vi "LabVIEW Final Project read.vi"() -> ()   [LabVIEW 2022 SP3]
uses:
  <vilib>/sound2/lvsound2.llb/Sampling Mode.ctl
  <vilib>/Analysis/2dsp.llb/Real FFT.vi
  <vilib>/Analysis/baseanly.llb/Mean (DBL).vi
  <vilib>/sound2/lvsound2.llb/Sound Input Read (DBL).vi
  <vilib>/measure/matone.llb/Extract Multiple Tone Information 1 Chan.vi
  <vilib>/Utility/file.llb/Read Delimited Spreadsheet (DBL).vi
  <vilib>/Analysis/NI_AALPro.lvlib
  <vilib>/measure/NI_MAPro.lvlib
  <vilib>/Analysis/NI_AALBase.lvlib
panel:
  in  "stop":bool
  out "Average Percent Difference from Phase":dbl
  out "Average Percent Difference from Frequency":dbl
  out "Average Percent Difference from Amplitude":dbl format="%#_10g"
  out "On if same voice, Off if different":bool
  out "multiple tone information":T1(array[cluster]) {"detected phase (deg)" format="%_6g"; "detected amplitude" format="%_6p"; "detected frequency" format="%_6p"}
  out "Spectrum":dbl[](graph)
  out "Original":dbl[](graph)
  in  "Press to take input":bool
  # "Now I need to change Sensitivity Values"
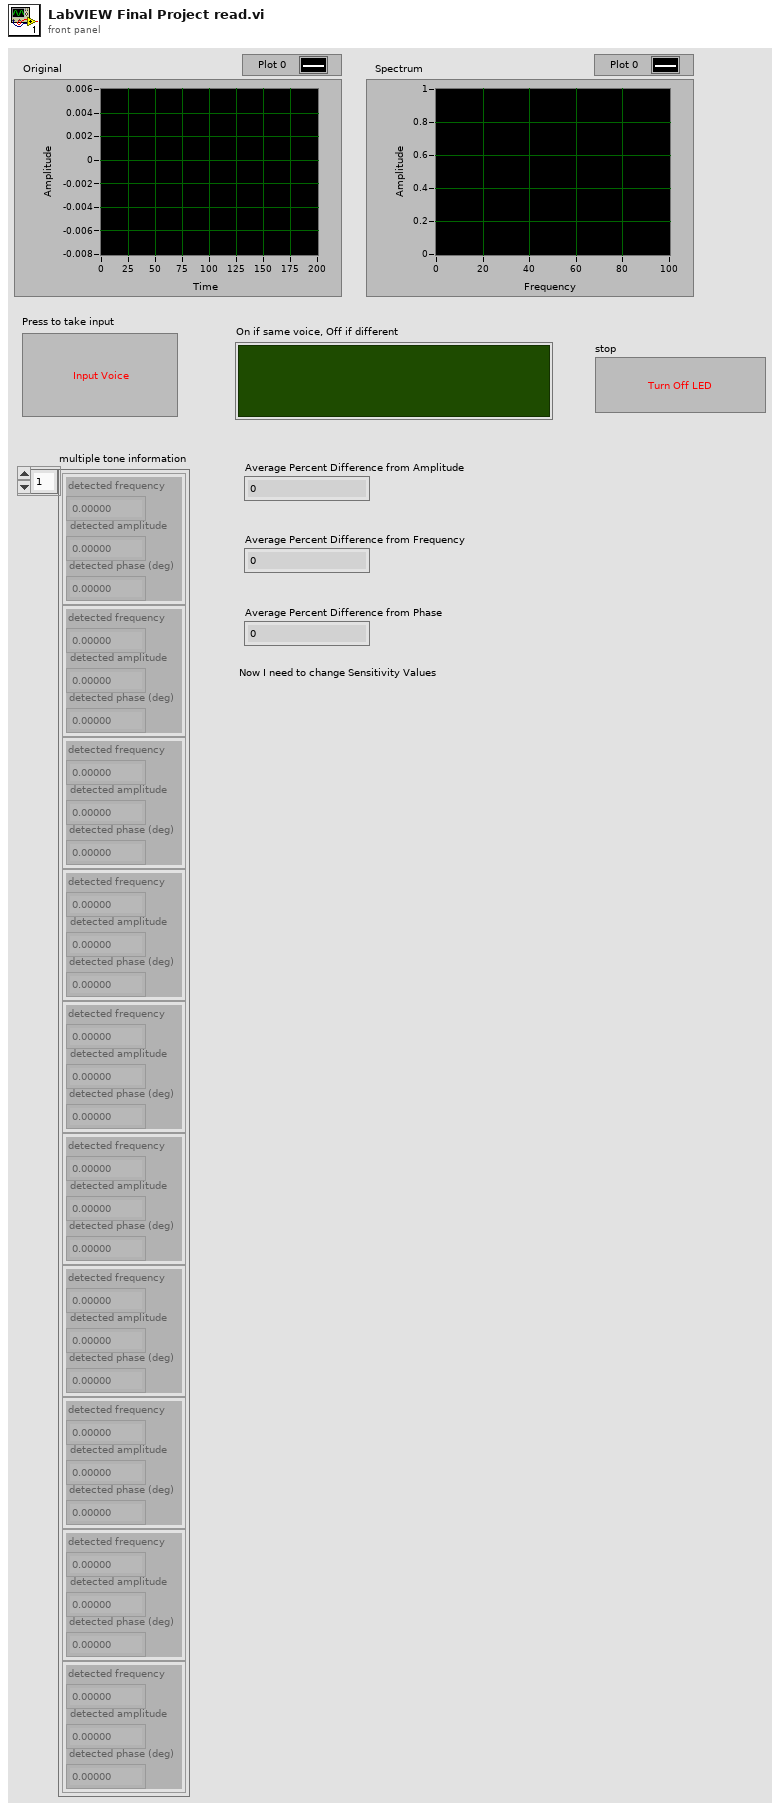
[diagram p1: front panel]
types:
  T1 = cluster{"detected frequency":dbl, "detected amplitude":dbl, "detected phase (deg)":dbl}[]
  T2 = enum32{"none", "input signal", "detected signal", "residual signal"}
  T3 = typedef "Sampling Mode.ctl" = i32
  T4 = typedef "Sound Input Task ID.ctl" = u32
  T5 = cluster{"detected frequency":dbl, "detected amplitude":dbl, "detected phase (deg)":dbl}
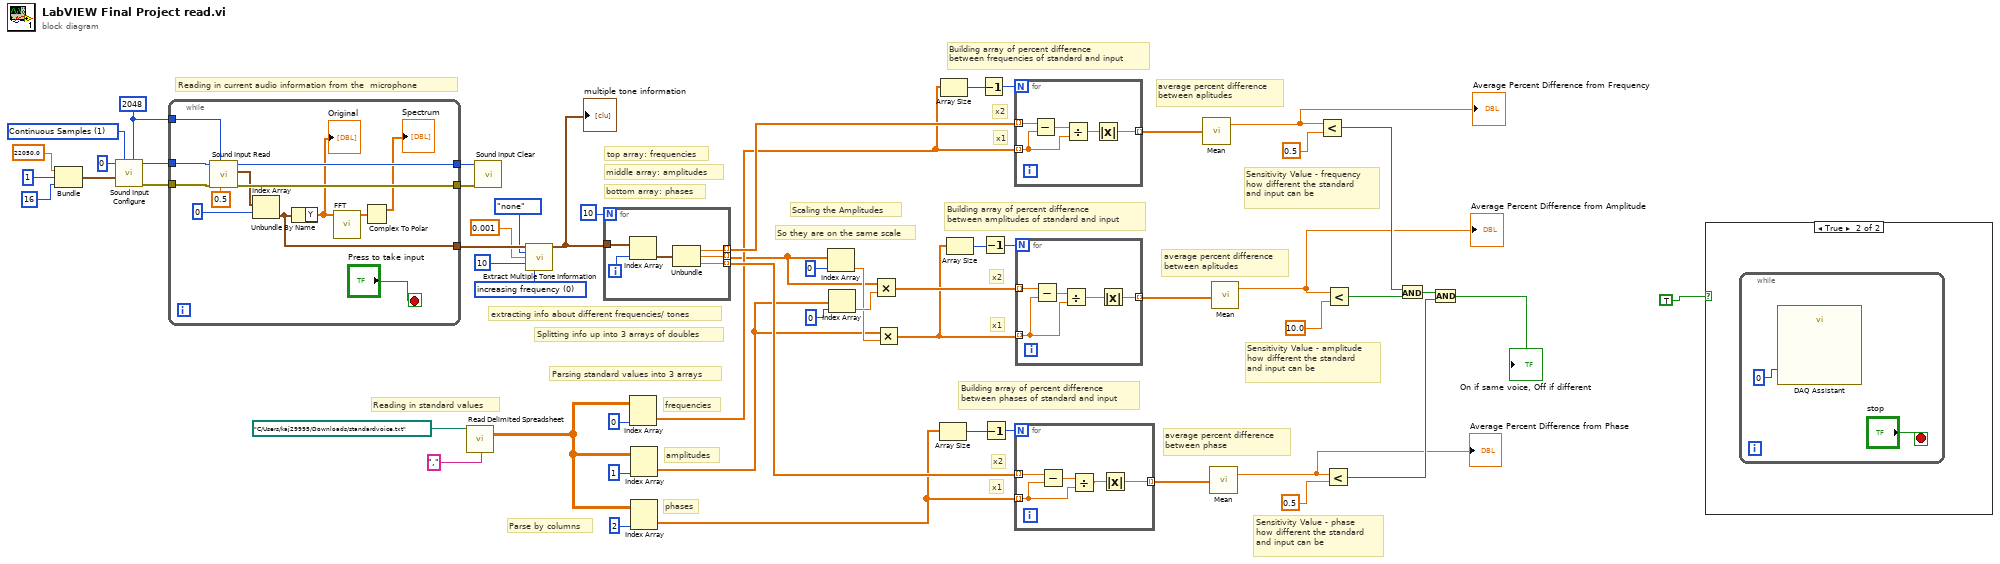
[diagram p0: block diagram]
diagram:
  w40 = 0 items=["increasing frequency", "decreasing amplitude"] ("output sorting")
  w49 = 2048 ("number of samples/ch")
  w52 = T3 1 items=["Finite Samples", "Continuous Samples"] ("sample mode")
  # "Parse by columns"
  # "Sensitivity Value - phase\nhow different the standard \nand input can be"
  # "average percent difference\nbetween phase"
  # "x2"
  # "x1"
  # "average percent difference\nbetween aplitudes"
  # "Sensitivity Value - frequency\nhow different the standard \nand input can be"
  # "x2"
  # "x1"
  # "Sensitivity Value - amplitude\nhow different the standard \nand input can be"
  # "average percent difference\nbetween aplitudes"
  # "x1"
  # "x2"
  # "Building array of percent difference \nbetween phases of standard and input"
  # "Building array of percent difference \nbetween frequencies of standard and input"
  # "Building array of percent difference \nbetween amplitudes of standard and input"
  # "So they are on the same scale"
  # "Splitting info up into 3 arrays of doubles"
  # "extracting info about different frequencies/ tones"
  # "Reading in current audio information from the  microphone"
  # "bottom array: phases"
  # "middle array: amplitudes"
  # "top array: frequencies"
  # "phases"
  # "amplitudes"
  # "frequencies"
  # "Parsing standard values into 3 arrays"
  # "Reading in standard values"
  # "Scaling the Amplitudes"
  n1 = Bundle(22050.0, 1, 16) -> (w54:cluster{dbl, i32, i32})  [unwired: 1 in]
  n2 = call <vilib>:"Sound Input Configure.vi"("number of samples/ch"=w49, "sample mode"=w52, "sound format"=w54, "device ID"=u32 0) -> ("error out"=w51:errorcluster, "task ID"=w50:T4)  [unwired: 6 in]
  n3 = while {
    tunnel: w51 -> [w67]
    tunnel: w50 -> [w66]
    tunnel: w49 -> [w65]
    tunnel: [w64] -> w48
    tunnel: [w63] -> w47
    tunnel: [w58] -> w44
    stop <- "Press to take input" stop-if-true
    n4 = call-poly <vilib>:"Sound Input Read.vi"("timeout (sec)"=0.5, "number of samples/ch"=w65, "error in (no error)"=w67, "task ID"=w66) -> ("error out"=w63:errorcluster, "data"=w60:waveform(dbl)[], "task ID out"=w64:T4)  [unwired: 5 in]
    n5 = Index Array(array=w60, index=0) -> (element=w58:waveform(dbl))
    n6 = Unbundle By Name(w58) -> ("Y"=w62:dbl[])
    "Original" <- w62
    n7 = call-poly <vilib>:"FFT.vi"("X"=w62) -> ("FFT {X}"=w61:cdb[])  [unwired: 9 in, 1 out]
    n8 = Complex To Polar(r * e^(i*theta)=w61) -> (r=→"Spectrum":dbl[])  [unwired: 1 out]
  }
  n9 = call-poly <vilib>:"Read Delimited Spreadsheet.vi"("file path (dialog if empty)"=path "C:/Users/kaj29995/Downloads/standardvoice.txt" ("file (use dialog)"), "delimiter (\\t)"=",") -> ("all rows"=w12:dbl[][])  [unwired: 8 in, 5 out]
  n10 = call <vilib>:"Sound Input Clear.vi"("error in (no error)"=w47, "task ID"=w48) -> ()  [unwired: 9 in, 1 out]
  n11 = call-poly <vilib>:"Extract Multiple Tone Information.vi"("time signal in"=w44, "export mode"=T2."none", "threshold"=0.001, "max num tones"=10, "output sorting"=w40) -> ("multiple tone information"=w45:T1)  [unwired: 8 in, 2 out]
  "multiple tone information" <- w45
  n12 = for {
    N: 10 -> [_]
    tunnel: w45 -> [w76]
    tunnel: [w71] -> w5 mode=indexing
    tunnel: [w73] -> w35 mode=indexing
    tunnel: [w72] -> w34 mode=indexing
    i -> [w74]
    n13 = Index Array(array=w76, index=w74) -> (element=w75:T5)
    n14 = Unbundle(w75) -> ("detected frequency"=w73:dbl, "detected amplitude"=w71:dbl, "detected phase (deg)"=w72:dbl)
  }
  n15 = Index Array(array=w12, index (col)=0 ("disabled index (col)")) -> (element=w11:dbl[])  [unwired: 1 in]
  n16 = Index Array(array=w12, index (col)=1 ("disabled index (col)")) -> (element=w10:dbl[])  [unwired: 1 in]
  n17 = Index Array(array=w12, index (col)=2 ("disabled index (col)")) -> (element=w9:dbl[])  [unwired: 1 in]
  n18 = Index Array(array=w5, index=0) -> (element=w36:dbl)
  n19 = Index Array(array=w10, index=0) -> (element=w37:dbl)
  n20 = Multiply(x=w5, y=w37) -> (x*y=w33:dbl[])
  n21 = Multiply(x=w10, y=w36) -> (x*y=w8:dbl[])
  n22 = Array Size(array=w9) -> (size(s)=w25:i32)
  n23 = Array Size(array=w11) -> (size(s)=w29:i32)
  n24 = Array Size(array=w8) -> (size(s)=w7:i32)
  n25 = Decrement(x=w29) -> (x-1=w4:i32)
  n26 = Decrement(x=w7) -> (x-1=w6:i32)
  n27 = Decrement(x=w25) -> (x-1=w3:i32)
  n28 = for {
    N: w4 -> [_]
    tunnel: w35 -> [w81] mode=indexing
    tunnel: w11 -> [w79] mode=indexing
    tunnel: [w77] -> w28 mode=indexing
    n29 = Subtract(x=w81, y=w79) -> (x-y=w80:dbl)
    n30 = Divide(x=w80, y=w79) -> (x/y=w78:dbl)
    n31 = Absolute Value(x=w78) -> (abs(x)=w77:dbl)
  }
  n32 = for {
    N: w3 -> [_]
    tunnel: w34 -> [w85] mode=indexing
    tunnel: w9 -> [w84] mode=indexing
    tunnel: [w82] -> w24 mode=indexing
    n33 = Subtract(x=w85, y=w84) -> (x-y=w86:dbl)
    n34 = Divide(x=w86, y=w84) -> (x/y=w83:dbl)
    n35 = Absolute Value(x=w83) -> (abs(x)=w82:dbl)
  }
  n36 = for {
    N: w6 -> [_]
    tunnel: w33 -> [w90] mode=indexing
    tunnel: w8 -> [w87] mode=indexing
    tunnel: [w88] -> w18 mode=indexing
    n37 = Subtract(x=w90, y=w87) -> (x-y=w91:dbl)
    n38 = Divide(x=w91, y=w87) -> (x/y=w89:dbl)
    n39 = Absolute Value(x=w89) -> (abs(x)=w88:dbl)
  }
  n40 = call-poly <vilib>:"Mean.vi"("X"=w28) -> ("mean"=w20:dbl)  [unwired: 1 out]
  "Average Percent Difference from Frequency" <- w20
  n41 = call-poly <vilib>:"Mean.vi"("X"=w24) -> ("mean"=w19:dbl)  [unwired: 1 out]
  "Average Percent Difference from Phase" <- w19
  n42 = call-poly <vilib>:"Mean.vi"("X"=w18) -> ("mean"=w21:dbl)  [unwired: 1 out]
  "Average Percent Difference from Amplitude" <- w21
  n43 = Less?(x=w20, y=0.5) -> (x < y?=w26:bool)
  n44 = Less?(x=w19, y=0.5) -> (x < y?=w22:bool)
  n45 = Less?(x=w21, y=10.0) -> (x < y?=w31:bool)
  n46 = And(x=w26, y=w31) -> (x .and. y?=w30:bool)
  n47 = And(x=w30, y=w22) -> (x .and. y?=→"On if same voice, Off if different":bool)
  n48 = case shown="True" TRUE {
    frame False {
    }
    frame True {
      n49 = while {
        stop <- "stop" stop-if-true
        n50 = call "DAQ Assistant"("data"=0) -> ()  [unwired: 17 in, 2 out]
      }
    }
  }
